vi "Edit Mail Steptypes.vi"(8 "error in":errorcluster, 10 "Mail In":T1={"Configure Server"={"Outgoing Mail Server (SMTP)"="smtp.gmail.com", "Port"="587", "Sender's Email Address"="ltt24012025@gmail.com", "username"="ltt24012025@gmail.com", "password"="hhib mwaf mimz fohz", "Enable TLS"=TRUE}, "Data"={"Subject"="", "Message"="", "TO"=[], "CC"=[]}, "Sent"=FALSE, "MAIL Operation"=enum."Init"}, 11 "Sequence Context In":refnum<k7>) -> (0 "error out":errorcluster, 2 "Mail Out":T1={"Configure Server"={"Outgoing Mail Server (SMTP)"="smtp.gmail.com", "Port"="587", "Sender's Email Address"="ltt24012025@gmail.com", "username"="ltt24012025@gmail.com", "password"="hhib mwaf mimz fohz", "Enable TLS"=TRUE}, "Data"={"Subject"="", "Message"="", "TO"=[], "CC"=[]}, "Sent"=FALSE, "MAIL Operation"=enum."Init"})   [LabVIEW 2023, in "LTT_TeststandSteptypes.lvlib"]
uses:
  LTT_TeststandSteptypes.lvlib
  Control/Configure Mail Setting.ctl
  Control/Mail Message Data.ctl
  Control/Mail Data.ctl
  <vilib>/addons/TestStand/_TSUtility.llb/TestStand - Start Modal Dialog (Sequence Context).vi
  <vilib>/addons/TestStand/_TSUtility.llb/TestStand - End Modal Dialog (Sequence Context).vi
panel:
  in  "MAIL Operation":enum32{"Init", "Configure", "Sent", "Close"}(tab)
  in  "Configure Server":T2={"Outgoing Mail Server (SMTP)"="smtp.gmail.com", "Port"="587", "Sender's Email Address"="ltt24012025@gmail.com", "username"="ltt24012025@gmail.com", "password"="hhib mwaf mimz fohz", "Enable TLS"=TRUE}
  in  "Data":T3
  in  "Mail Enable":bool
  in  "Close":bool
  in  "OK":bool
  # "Mail Reference it close"
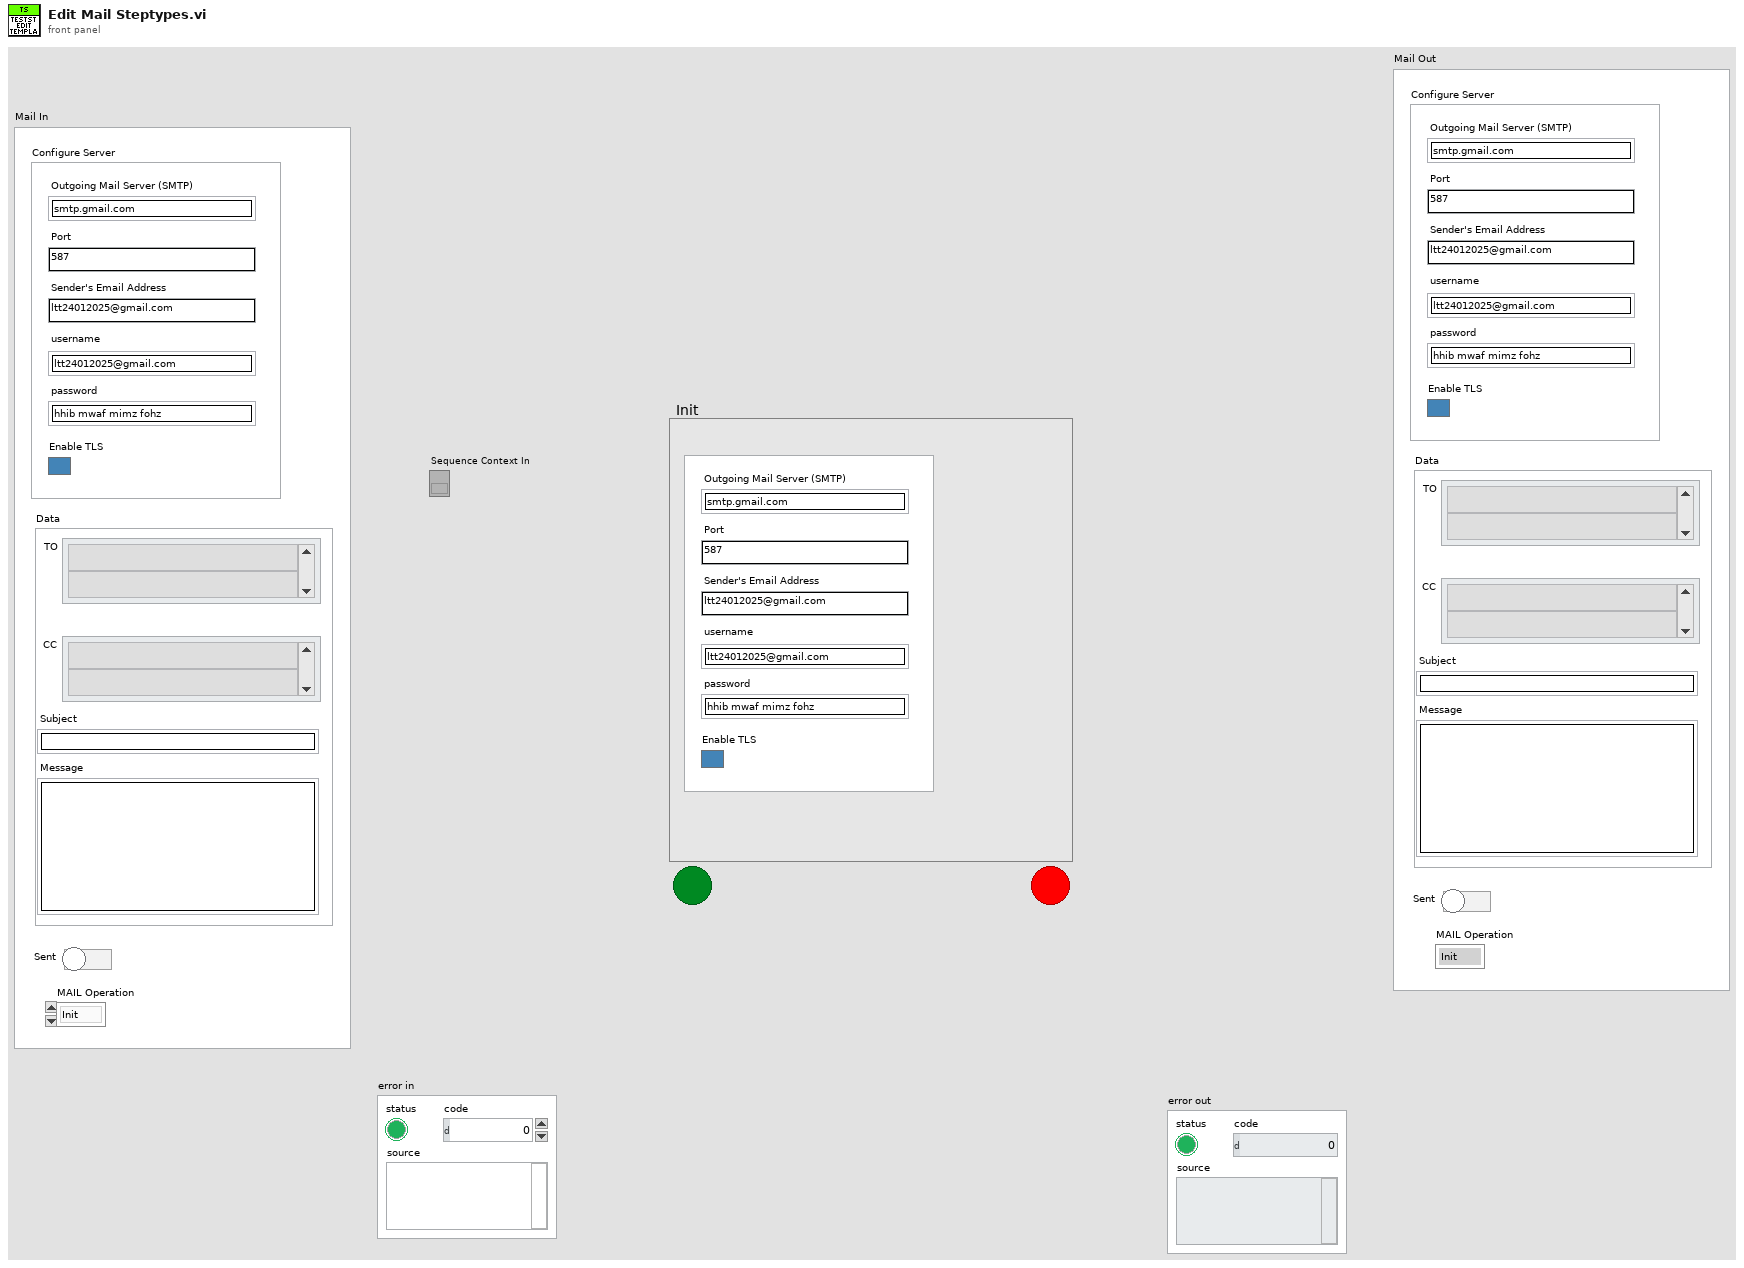
[diagram p1: front panel]
types:
  T1 = typedef "LTT_TeststandSteptypes.lvlib/Mail Data.ctl" = cluster{"Configure Server":T2, "Data":T3, "Sent":bool, "MAIL Operation":enum32{"Init", "Configure", "Sent", "Close"}}
  T2 = typedef "LTT_TeststandSteptypes.lvlib/Configure Mail Setting.ctl" = cluster{"Outgoing Mail Server (SMTP)":string, "Port":string, "Sender's Email Address":string, "username":string, "password":string, "Enable TLS":bool}
  T3 = typedef "LTT_TeststandSteptypes.lvlib/Mail Message Data.ctl" = cluster{"Subject":string, "Message":string, "TO":string[], "CC":string[]}
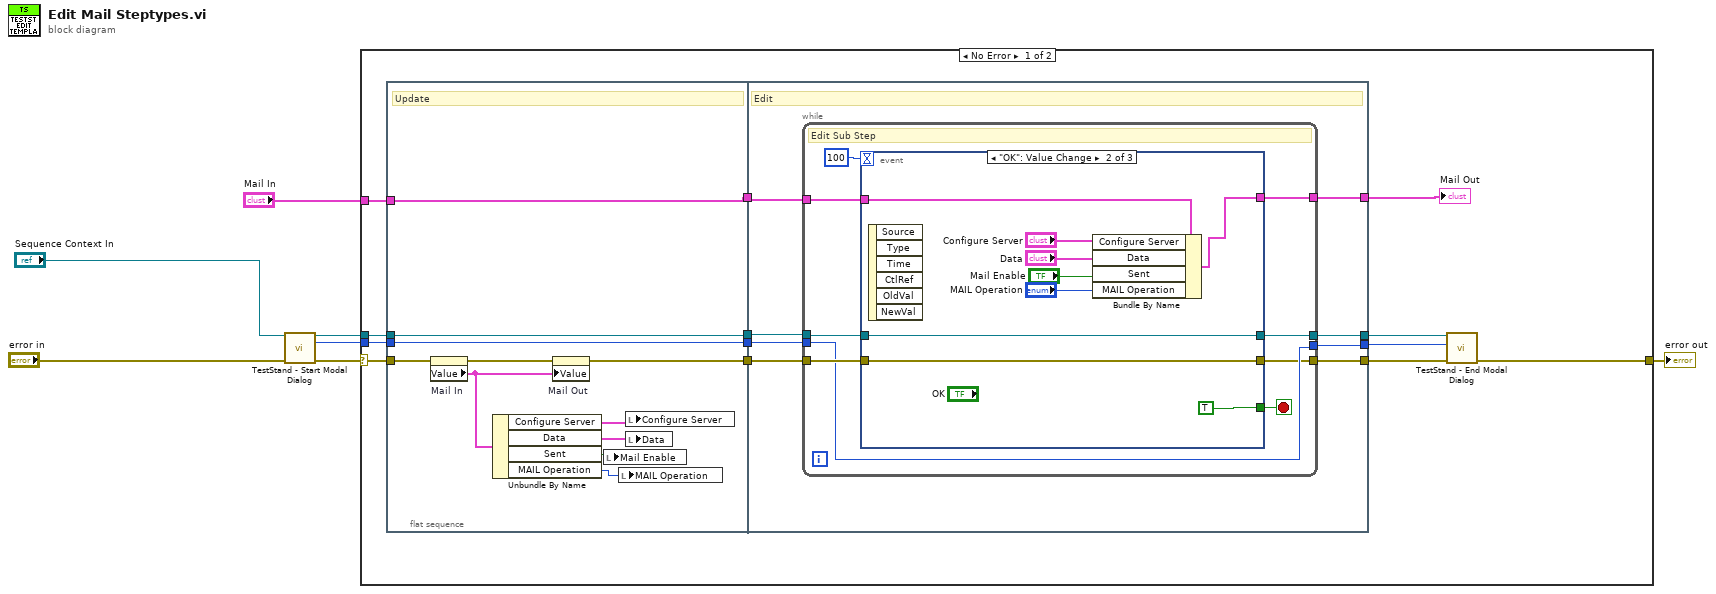
[diagram p0: block diagram]
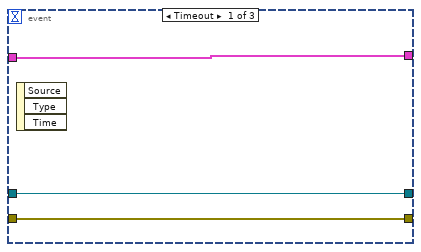
[diagram p2: hidden frame]
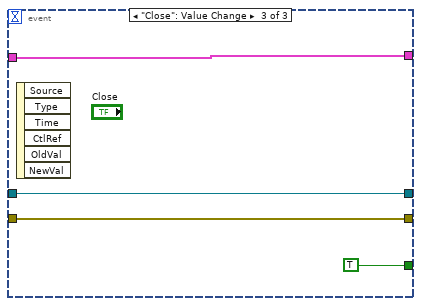
[diagram p3: hidden frame]
diagram:
  n1 = call-poly <vilib>:"TestStand - Start Modal Dialog.vi"("Sequence Context In"="Sequence Context In", "error in (no error)"="error in") -> ("Sequence Context Out"=w5:refnum<k7>, "Modal ID"=w4:i32, "error out"=w6:errorcluster)  [unwired: 9 in, 2 out]
  n2 = case shown="No Error" w6 {
    selector: w6 -> [w17 w65]
    tunnel: w5 -> [w15 _]
    tunnel: w4 -> [w14 _]
    tunnel: [w11 w65] -> w3
    tunnel: "Mail In" -> [w9 _]
    frame No Error {
      n3 = flat-sequence {
        tunnel: w17 -> [w29]
        tunnel: [w27] -> w20
        tunnel: w15 -> [w31]
        tunnel: w14 -> [w30]
        tunnel: [w31] -> w19
        tunnel: [w30] -> w18
        tunnel: [w26] -> w10
        tunnel: w9 -> [w26]
        tunnel: w20 -> [w37]
        tunnel: [w35] -> w16
        tunnel: w19 -> [w39]
        tunnel: w18 -> [w38]
        tunnel: [w36] -> w13
        tunnel: [w34] -> w12
        tunnel: w10 -> [w33]
        tunnel: [w32] -> w8
        frame #0 {
          # "Update"
          n4 = property on="Mail In" class="Clust (strict)"(error in=w29) -> (error out=w28:errorcluster, "Value"=w25:T1)  [unwired: 1 in, 1 out]
          n5 = Unbundle By Name(w25) -> ("Configure Server"=w24:T2, "Data"=w23:T3, "Sent"=w21:bool, "MAIL Operation"=w22:enum32{"Init", "Configure", "Sent", "Close"})
          n6 = property on="Mail Out" class="Clust (strict)"(error in=w28, "Value"=w25) -> (error out=w27:errorcluster)  [unwired: 1 in, 1 out]
          n7 = local write "Mail Enable"(w21) -> ()
          n8 = local write "MAIL Operation"(w22) -> ()
          n9 = local write "Configure Server"(w24) -> ()
          n10 = local write "Data"(w23) -> ()
        }
        frame #1 {
          # "Edit"
          n11 = while {
            tunnel: w39 -> [w46]
            tunnel: w38 -> [w43]
            tunnel: w37 -> [w44]
            tunnel: [w45] -> w34
            tunnel: [w43] -> w36
            tunnel: [w42] -> w35
            tunnel: w33 -> [w41]
            tunnel: [w40] -> w32
            stop <- w47 stop-if-true
            # "Edit Sub Step"
            n12 = event shown="[1] \"OK\": Value Change" {
              selector: _ -> [_ _ _]
              dyn-events: _ -> [_ _ _]
              timeout: 100 -> [_ _ _]
              tunnel: [_ TRUE TRUE] -> w47
              tunnel: [w50 w58 w63] -> w45
              tunnel: w46 -> [w50 w58 w63]
              tunnel: w44 -> [w49 w59 w62]
              tunnel: [w49 w59 w62] -> w42
              tunnel: w41 -> [w51 w57 w61]
              tunnel: [w51 w56 w61] -> w40
              event Timeout {
                n13 = event-data() -> ()  [unwired: 1 in, 3 out]
              }
              event "OK": Value Change {
                n14 = event-data() -> ()  [unwired: 1 in, 6 out]
                n15 = Bundle By Name(cluster=w57, "Configure Server"="Configure Server", "Data"="Data", "Sent"="Mail Enable", "MAIL Operation"="MAIL Operation") -> (w56:T1)
              }
              event "Close": Value Change {
                n16 = event-data() -> ()  [unwired: 1 in, 6 out]
              }
            }
          }
        }
      }
      n17 = call-poly <vilib>:"TestStand - End Modal Dialog.vi"("Sequence Context In"=w12, "Modal ID"=w13, "error in (no error)"=w16) -> ("error out"=w11:errorcluster)  [unwired: 12 in]
      "Mail Out" <- w8
    }
    frame Error {
    }
  }
  "error out" <- w3
